vi "WPI_ServoSetAngle.vi"(8 "error in (no error)":errorcluster, 10 "Angle":i32, 11 "ServoDeviceRef":T1={"DeviceStatus"={"status"=FALSE, "code"=0, "source"=""}, "PWM Channel"=enum."Invalid", "DeadBand"={"Name"="", "maxPositivePwm"=0, "minPositivePwm"=0, "centerPwm"=0, "maxNegativePwm"=0, "minNegativePwm"=0, "angularRange"=0}}) -> (0 "error out":errorcluster, 3 "ServoDeviceRef":T1={"DeviceStatus"={"status"=FALSE, "code"=0, "source"=""}, "PWM Channel"=enum."Invalid", "DeadBand"={"Name"="", "maxPositivePwm"=0, "minPositivePwm"=0, "centerPwm"=0, "maxNegativePwm"=0, "minNegativePwm"=0, "angularRange"=0}})   [LabVIEW 2017]
doc: "Sets the angle of the servo you specify.\n\nThis software is licensed. Open the labview\\readme\\WPI Robotics Library Open Source License.txt file for more information."
uses:
  <vilib>/Rock Robotics/WPI/PWM/Servo/WPI_ServoDeviceRef.ctl
  <vilib>/Rock Robotics/SystemInterfaces/DIO/FPGA_DIOPWMChannel.ctl
  <vilib>/Rock Robotics/WPI/PWM/WPI_PWMDeadband.ctl
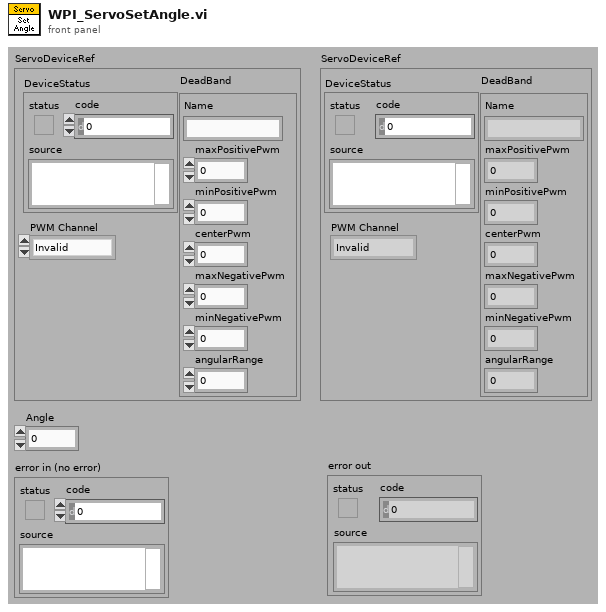
[diagram p1: front panel]
types:
  T1 = typedef "WPI_ServoDeviceRef.ctl" = cluster{"DeviceStatus":errorcluster, "PWM Channel":T2, "DeadBand":T3}
  T2 = typedef "FPGA_DIOPWMChannel.ctl" = enum8{"PWM 0", "PWM 1", "PWM 2", "PWM 3", "PWM 4", "PWM 5", "PWM 6", "PWM 7", "PWM 8", "PWM 9", "PWM MXP 0", "PWM MXP 1", "PWM MXP 2", "PWM MXP 3", "PWM MXP 4", "PWM MXP 5", "PWM MXP 6", "PWM MXP 7", "PWM MXP 8", "PWM MXP 9", "Invalid"}
  T3 = typedef "WPI_PWMDeadband.ctl" = cluster{"Name":string, "maxPositivePwm":i32, "minPositivePwm":i32, "centerPwm":i32, "maxNegativePwm":i32, "minNegativePwm":i32, "angularRange":u16}
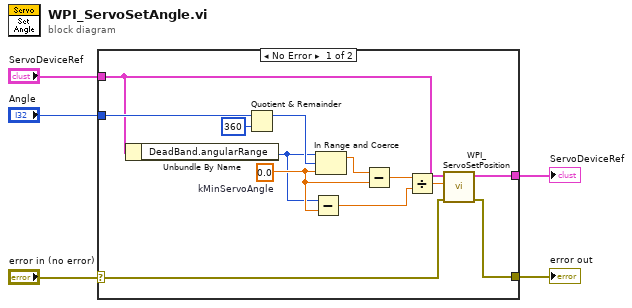
[diagram p0: block diagram]
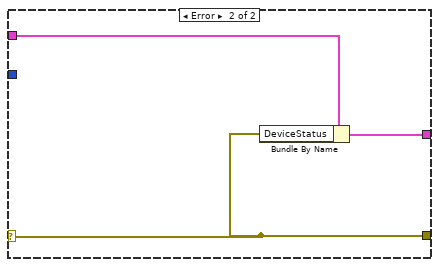
[diagram p2: hidden frame]
diagram:
  n1 = case shown="No Error" "error in (no error)" {
    selector: "error in (no error)" -> [w18 w19]
    tunnel: "ServoDeviceRef" -> [w6 w21]
    tunnel: [w17 w20] -> w4
    tunnel: "Angle" -> [w15 _]
    tunnel: [w16 w19] -> w2
    frame No Error {
      w12 = 0.0  # kMinServoAngle
      n2 = Unbundle By Name(w6) -> ("DeadBand.angularRange"=w7:u16)
      n3 = Quotient & Remainder(x=w15, y=360) -> (x-y*floor(x/y)=w8:i32)  [unwired: 1 out]
      n4 = Subtract(x=w7, y=w12) -> (x-y=w10:dbl)
      n5 = In Range and Coerce(upper limit=w7, x=w8, lower limit=w12) -> (coerced(x)=w13:dbl)  [unwired: 1 out]
      n6 = Subtract(x=w13, y=w12) -> (x-y=w11:dbl)
      n7 = Divide(x=w11, y=w10) -> (x/y=w9:dbl)
      n8 = call <vilib>:"WPI_ServoSetPosition.vi"("error in (no error)"=w18, "Position"=w9, "ServoDeviceRef"=w6) -> ("error out"=w16:errorcluster, "ServoDeviceRef"=w17:T1)  [unwired: 7 out]
    }
    frame Error {
      n9 = Bundle By Name(cluster=w21, "DeviceStatus"=w19) -> (w20:T1)
    }
  }
  "ServoDeviceRef" <- w4
  "error out" <- w2
